vi "SetZone.vi"(4 "AttackingOurselves":bool, 6 "ZoneParameters":T1, 8 "error in (no error)":errorcluster, 9 "Enum":T2, 10 "Field":refnum<class "Field.lvclass">, 11 "object in":refnum<class "Zone.lvclass">) -> (0 "error out":errorcluster, 3 "object out":refnum<class "Zone.lvclass">)   [LabVIEW 2023, in "Zone.lvclass"]
uses:
  Zone.lvclass
  zones.ctl
  Field_class/Field.lvclass
  Zone.lvclass/Zone.ctl
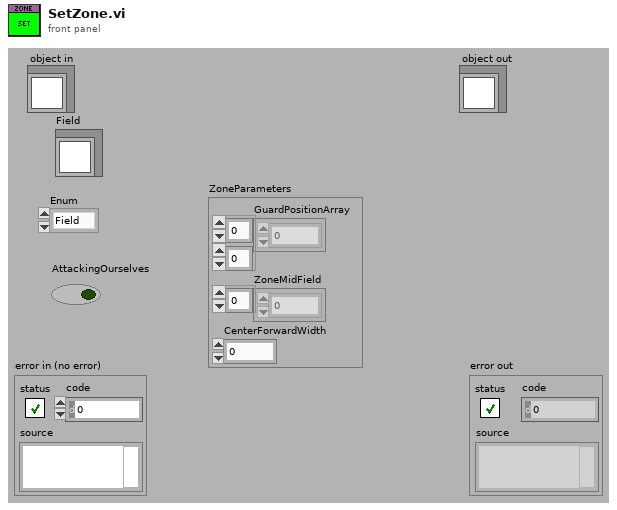
[diagram p1: front panel]
types:
  T1 = cluster{"GuardPositionArray":dbl[][], "ZoneMidField":dbl[], "CenterForwardWidth":dbl}
  T2 = typedef "Zone.lvclass/zones.ctl" = enum16{"Field", "LeftSide", "RightSide", "MidField", "LeftForward", "RightForward", "LeftMidField", "RightMidField", "LeftWing", "CenterForward", "RightWing", "Size"}
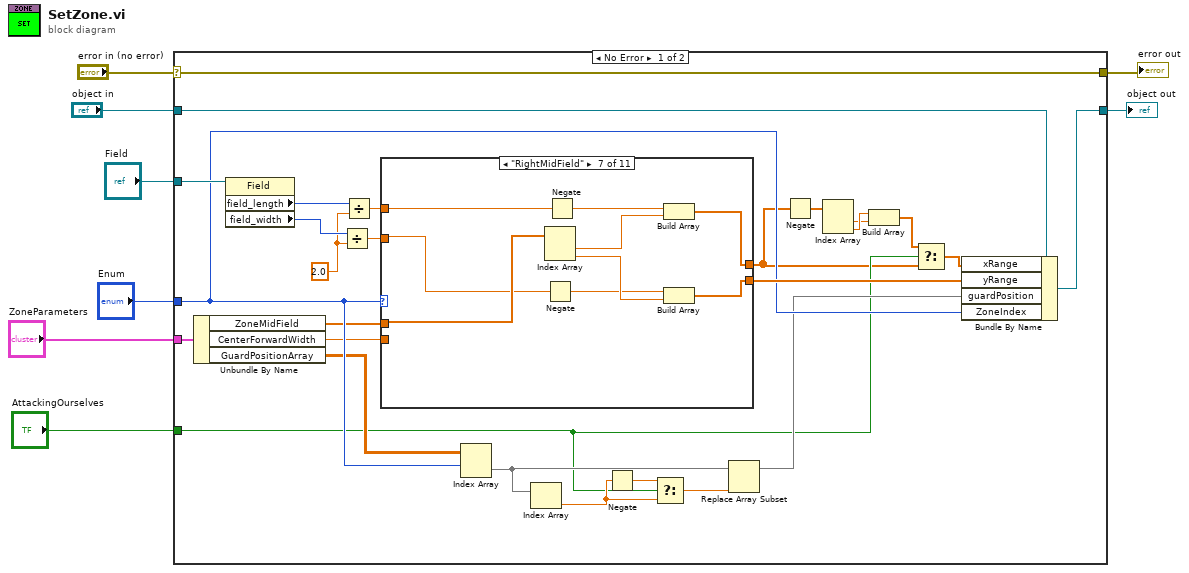
[diagram p0: block diagram]
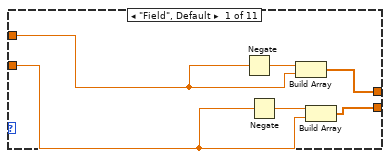
[diagram p2: hidden frame]
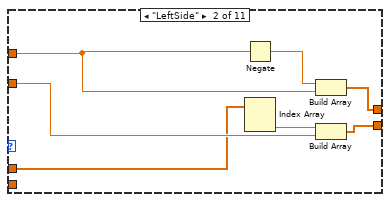
[diagram p3: hidden frame]
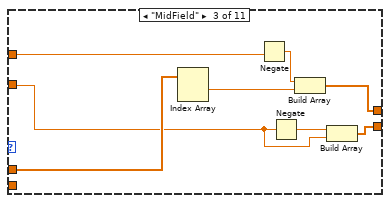
[diagram p4: hidden frame]
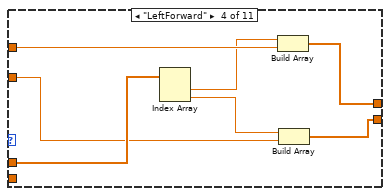
[diagram p5: hidden frame]
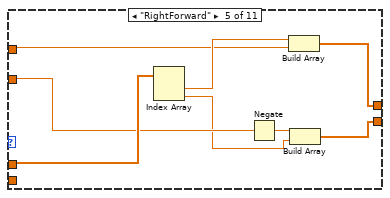
[diagram p6: hidden frame]
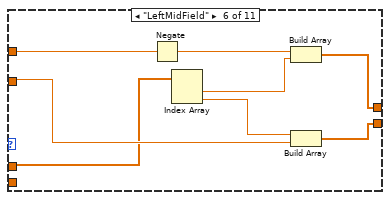
[diagram p7: hidden frame]
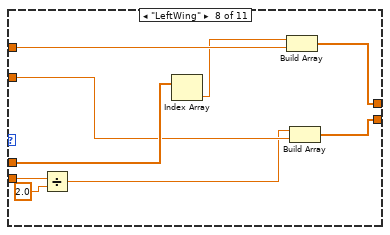
[diagram p8: hidden frame]
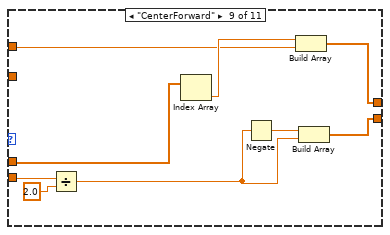
[diagram p9: hidden frame]
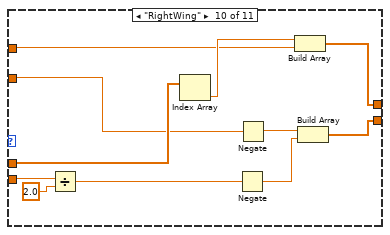
[diagram p10: hidden frame]
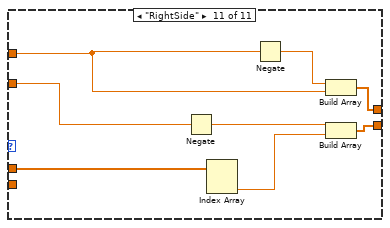
[diagram p11: hidden frame]
diagram:
  n1 = case shown="No Error" "error in (no error)" {
    selector: "error in (no error)" -> [w35 w127]
    tunnel: [w35 w127] -> w7
    tunnel: [w33 w126] -> w5
    tunnel: "object in" -> [w34 w126]
    tunnel: "Enum" -> [w24 _]
    tunnel: "Field" -> [w32 _]
    tunnel: "ZoneParameters" -> [w25 _]
    tunnel: "AttackingOurselves" -> [w15 _]
    frame No Error {
      w30 = 2.0 ("y")
      n2 = Unbundle By Name(w25) -> ("ZoneMidField"=w16:dbl[], "CenterForwardWidth"=w17:dbl, "GuardPositionArray"=w18:dbl[][])
      n3 = property class="Field"(reference=w32) -> ("field_length"=w29:i32, "field_width"=w31:i32)  [unwired: 1 in, 2 out]
      n4 = Divide(x=w31, y=w30) -> (x/y=w27:dbl)
      n5 = Divide(x=w29, y=w30) -> (x/y=w28:dbl)
      n6 = case shown="\"RightMidField\"" w24 {
        tunnel: w28 -> [w38 w47 w55 w62 w70 w76 w86 w97 w104 w115 w124]
        tunnel: w27 -> [w36 w46 w49 w58 w68 w78 w81 w94 _ w110 w122]
        tunnel: [w40 w45 w52 w63 w64 w73 w84 w89 w99 w112 w119] -> w10
        tunnel: [w39 w44 w51 w57 w65 w72 w83 w90 w98 w111 w120] -> w26
        tunnel: w17 -> [_ _ _ _ _ _ _ w93 w102 w113 _]
        tunnel: w16 -> [_ w43 w54 w61 w69 w77 w85 w95 w103 w114 w123]
        frame "Field", Default {
          n7 = Negate(x=w38) -> (-x=w41:dbl)
          n8 = Negate(x=w36) -> (-x=w37:dbl)
          n9 = Build Array(w41, w38) -> (w40:dbl[])
          n10 = Build Array(w37, w36) -> (w39:dbl[])
        }
        frame "LeftSide" {
          n11 = Negate(x=w47) -> (-x=w48:dbl)
          n12 = Index Array(array=w43) -> (element #2=w42:dbl)  [unwired: 2 in, 1 out]
          n13 = Build Array(w48, w47) -> (w45:dbl[])
          n14 = Build Array(w42, w46) -> (w44:dbl[])
        }
        frame "MidField" {
          n15 = Index Array(array=w54) -> (element #1=w53:dbl)  [unwired: 2 in, 1 out]
          n16 = Negate(x=w55) -> (-x=w56:dbl)
          n17 = Negate(x=w49) -> (-x=w50:dbl)
          n18 = Build Array(w56, w53) -> (w52:dbl[])
          n19 = Build Array(w50, w49) -> (w51:dbl[])
        }
        frame "LeftForward" {
          n20 = Index Array(array=w61) -> (element #1=w59:dbl, element #2=w60:dbl)  [unwired: 2 in]
          n21 = Build Array(w59, w62) -> (w63:dbl[])
          n22 = Build Array(w60, w58) -> (w57:dbl[])
        }
        frame "RightForward" {
          n23 = Index Array(array=w69) -> (element #1=w71:dbl, element #2=w66:dbl)  [unwired: 2 in]
          n24 = Negate(x=w68) -> (-x=w67:dbl)
          n25 = Build Array(w71, w70) -> (w64:dbl[])
          n26 = Build Array(w67, w66) -> (w65:dbl[])
        }
        frame "LeftMidField" {
          n27 = Negate(x=w76) -> (-x=w75:dbl)
          n28 = Index Array(array=w77) -> (element #1=w74:dbl, element #2=w79:dbl)  [unwired: 2 in]
          n29 = Build Array(w75, w74) -> (w73:dbl[])
          n30 = Build Array(w79, w78) -> (w72:dbl[])
        }
        frame "RightMidField" {
          n31 = Index Array(array=w85) -> (element #1=w87:dbl, element #2=w82:dbl)  [unwired: 2 in]
          n32 = Negate(x=w81) -> (-x=w80:dbl)
          n33 = Negate(x=w86) -> (-x=w88:dbl)
          n34 = Build Array(w88, w87) -> (w84:dbl[])
          n35 = Build Array(w80, w82) -> (w83:dbl[])
        }
        frame "LeftWing" {
          n36 = Divide(x=w93, y=2.0) -> (x/y=w91:dbl)
          n37 = Index Array(array=w95) -> (element=w96:dbl)  [unwired: 1 in]
          n38 = Build Array(w96, w97) -> (w89:dbl[])
          n39 = Build Array(w91, w94) -> (w90:dbl[])
        }
        frame "CenterForward" {
          n40 = Divide(x=w102, y=2.0) -> (x/y=w100:dbl)
          n41 = Index Array(array=w103) -> (element=w106:dbl)  [unwired: 1 in]
          n42 = Negate(x=w100) -> (-x=w101:dbl)
          n43 = Build Array(w106, w104) -> (w99:dbl[])
          n44 = Build Array(w101, w100) -> (w98:dbl[])
        }
        frame "RightWing" {
          n45 = Divide(x=w113, y=2.0) -> (x/y=w108:dbl)
          n46 = Index Array(array=w114) -> (element=w117:dbl)  [unwired: 1 in]
          n47 = Negate(x=w108) -> (-x=w107:dbl)
          n48 = Negate(x=w110) -> (-x=w109:dbl)
          n49 = Build Array(w117, w115) -> (w112:dbl[])
          n50 = Build Array(w109, w107) -> (w111:dbl[])
        }
        frame "RightSide" {
          n51 = Negate(x=w122) -> (-x=w121:dbl)
          n52 = Index Array(array=w123) -> (element #2=w118:dbl)  [unwired: 2 in, 1 out]
          n53 = Negate(x=w124) -> (-x=w125:dbl)
          n54 = Build Array(w125, w124) -> (w119:dbl[])
          n55 = Build Array(w121, w118) -> (w120:dbl[])
        }
      }
      n56 = Index Array(array=w18, index (row)=w24) -> (element=w23:dbl[])  [unwired: 1 in]
      n57 = Index Array(array=w23) -> (element=w21:dbl)  [unwired: 1 in]
      n58 = Negate(x=w21) -> (-x=w22:dbl)
      n59 = Select(t=w22, s=w15, f=w21) -> (s? t:f=w20:dbl)
      n60 = Replace Array Subset(array=w23, new element=w20) -> (w19:dbl[])  [unwired: 1 in]
      n61 = Negate(x=w10) -> (-x=w14:dbl[])
      n62 = Index Array(array=w14) -> (element #1=w12:dbl, element #2=w13:dbl)  [unwired: 2 in]
      n63 = Build Array(w13, w12) -> (w11:dbl[])
      n64 = Select(t=w11, s=w15, f=w10) -> (s? t:f=w9:dbl[])
      n65 = Bundle By Name(cluster=w34, "xRange"=w9, "yRange"=w26, "guardPosition"=w19, "ZoneIndex"=w24) -> (w33:refnum<class "Zone.lvclass">)
    }
    frame Error {
    }
  }
  "error out" <- w7
  "object out" <- w5
